vi "UI.vi"(8 "Error in":errorcluster, 11 "Divide in":refnum<class "Divide.lvclass">) -> (0 "error out":errorcluster, 3 "Divide out":refnum<class "Divide.lvclass">)   [LabVIEW 2020, in "Divide.lvclass"]
uses:
  Divide.lvclass
  C:/Users/khishore.kumar/Khishore/labview_tips_2024/src/Assignment 25/Arithmetic Operations/Arithmetic Operations.lvclass
  Typedefs/User event operations.ctl
  Arithmetic Operations.lvclass/Arithmetic Operations.ctl
  Accessors/Write/Write A.vi
  Accessors/Write/Write B.vi
  Accessors/Read/Read C.vi
  Accessors/Read/Read A.vi
  Accessors/Read/Read B.vi
  Simple calculator.lvlib
panel:
  out "C":dbl
  in  "B":dbl
  in  "A":dbl
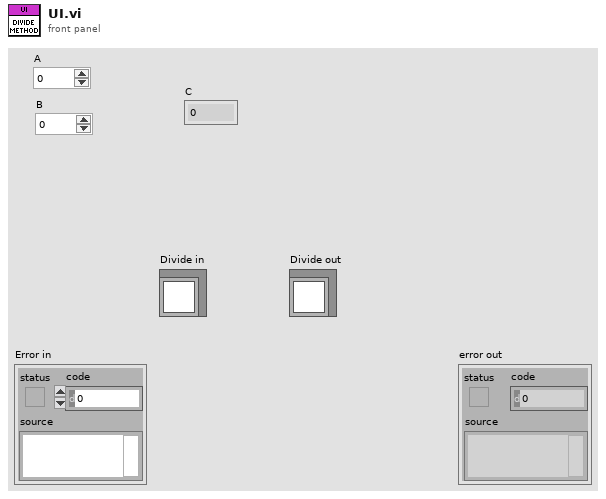
[diagram p1: front panel]
types:
  T1 = typedef "Simple calculator.lvlib/User event operations.ctl" = enum16{"Create", "Get Ref", "Generate ", "Destroy"}
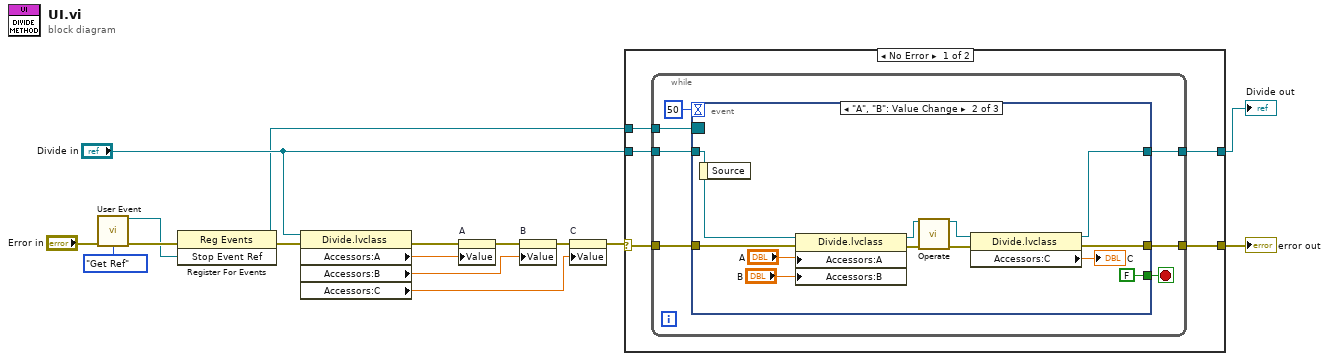
[diagram p0: block diagram]
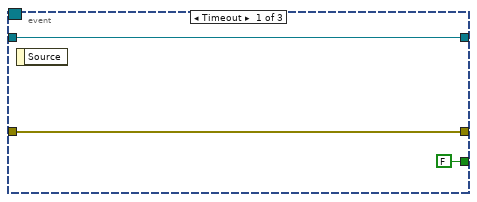
[diagram p2: hidden frame]
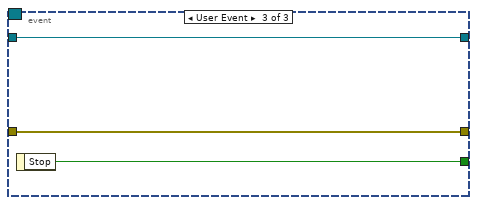
[diagram p3: hidden frame]
diagram:
  n1 = call "User Event.vi"("Error in"="Error in", "Operation"=User_event_operations."Get Ref") -> ("Stop Event Ref"=w14:refnum<user-event>, "Error out"=w15:errorcluster)  [unwired: 12 in]
  n2 = register-events(error in=w15, w14) -> (reference out=w1:refnum<event-registration>, error out=w11:errorcluster)  [unwired: 1 in]
  n3 = property class="Divide.lvclass"(reference="Divide in", error in=w11) -> (error out=w9:errorcluster, "Accessors:A"=w5:dbl, "Accessors:B"=w4:dbl, "Accessors:C"=w3:dbl)  [unwired: 1 out]
  n4 = property on="A" class="DigNum (strict)"(error in=w9, "Value"=w5) -> (error out=w8:errorcluster)  [unwired: 1 in, 1 out]
  n5 = property on="B" class="DigNum (strict)"(error in=w8, "Value"=w4) -> (error out=w7:errorcluster)  [unwired: 1 in, 1 out]
  n6 = property on="C" class="DigNum (strict)"(error in=w7, "Value"=w3) -> (error out=w6:errorcluster)  [unwired: 1 in, 1 out]
  n7 = case shown="No Error" w6 {
    selector: w6 -> [w19 w48]
    tunnel: [w20 w48] -> w16
    tunnel: "Divide in" -> [w21 w47]
    tunnel: [w18 w47] -> w2
    tunnel: w1 -> [w17 _]
    frame No Error {
      n8 = while {
        tunnel: w21 -> [w25]
        tunnel: [w28] -> w20
        tunnel: w19 -> [w27]
        tunnel: [w24] -> w18
        tunnel: w17 -> [w23]
        stop <- w22 stop-if-true
        n9 = event shown="[1] \"A\", \"B\": Value Change" {
          selector: w23 -> [_ _ _]
          dyn-events: _ -> [_ _ _]
          timeout: 50 -> [_ _ _]
          tunnel: [w31 w34 w45] -> w28
          tunnel: w27 -> [w31 w43 w45]
          tunnel: w25 -> [w30 w42 w44]
          tunnel: [w30 w33 w44] -> w24
          tunnel: [FALSE ("Stop") FALSE ("Stop") w46] -> w22
          event Timeout {
            n10 = event-data() -> ()  [unwired: 1 in, 1 out]
          }
          event "A", "B": Value Change {
            n11 = event-data() -> ()  [unwired: 1 in, 1 out]
            n12 = property class="Divide.lvclass"(reference=w42, error in=w43, "Accessors:A"="A", "Accessors:B"="B") -> (reference out=w38:refnum<class "Divide.lvclass">, error out=w39:errorcluster)
            n13 = call-dynamic "Operate.vi"("Divide in"=w38, "error in (no error)"=w39) -> ("Divide out"=w36:refnum<class "Divide.lvclass">, "error out"=w37:errorcluster)  [unwired: 12 in]
            n14 = property class="Divide.lvclass"(reference=w36, error in=w37) -> (reference out=w33:refnum<class "Divide.lvclass">, error out=w34:errorcluster, "Accessors:C"=→"C":dbl)
          }
          event User Event {
            n15 = event-data() -> ("Stop"=w46:bool)  [unwired: 1 in]
          }
        }
      }
    }
    frame Error {
    }
  }
  "error out" <- w16
  "Divide out" <- w2
